vi "Turn And Shoot.vi"(10 "Turning Angle":dbl, 11 "RobotDriveDevRef":T1) -> ()   [LabVIEW 2015]
uses:
  <vilib>/Rock Robotics/WPI/RobotDrive/WPI_RobotDriveArcadeDrive_Standard(NoSaturation).vi
  <vilib>/addons/control/pid/NI_PID_pid.lvlib
  <vilib>/addons/control/pid/pid.llb/PID (DBL).vi
  <vilib>/Rock Robotics/Network Tables/NT Read Number.vi
  <vilib>/Rock Robotics/Network Tables/NT Write Number.vi
  arm/arm.lvclass
  drive/drive.lvclass
  <vilib>/Rock Robotics/WPI/CAN/Jaguar/SubVIs/WPI_CANJaguar_ControlMode.ctl
  <vilib>/Rock Robotics/WPI/CAN/TalonSRX/WPI_CANTalonSRX_APIControlMode.ctl
  <vilib>/Rock Robotics/SystemInterfaces/DIO/FPGA_DIOPWMChannel.ctl
  <vilib>/Rock Robotics/WPI/PWM/WPI_PWMDeadband.ctl
  <vilib>/Rock Robotics/WPI/MotorControl/WPI_MotorControlType.ctl
  <vilib>/Rock Robotics/WPI/MotorControl/WPI_MotorControlDeviceRef.ctl
  <vilib>/Rock Robotics/WPI/RobotDrive/WPI_RobotDriveDevRef.ctl
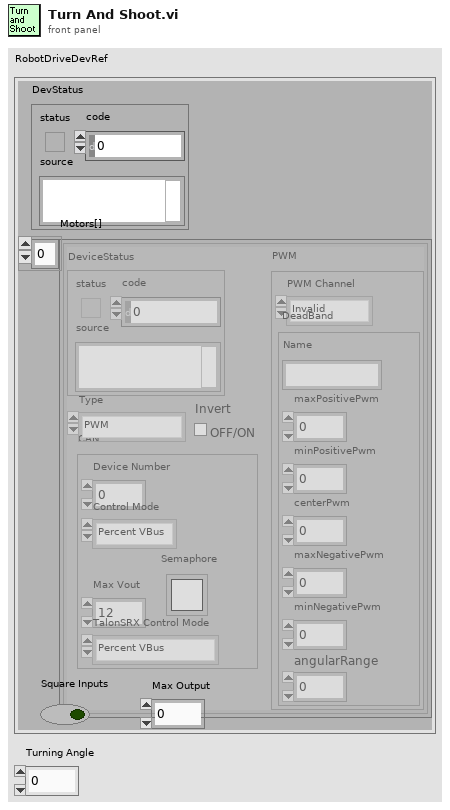
[diagram p1: front panel]
types:
  T1 = typedef "WPI_RobotDriveDevRef.ctl" = cluster{"DevStatus":errorcluster, "Motors[]":T2[], "Square Inputs":bool, "Max Output":dbl}
  T2 = typedef "WPI_MotorControlDeviceRef.ctl" = cluster{"DeviceStatus":errorcluster, "Type":T3, "PWM":cluster{"PWM Channel":T4, "DeadBand":T5}, "CAN":cluster{"Device Number":u8, "Control Mode":T6, "Semaphore":T7, "Max Vout":dbl, "TalonSRX Control Mode":T8}, "Invert":bool}
  T3 = typedef "WPI_MotorControlType.ctl" = enum16{"PWM", "CAN", "CANTalonSRX"}
  T4 = typedef "FPGA_DIOPWMChannel.ctl" = enum8{"PWM 0", "PWM 1", "PWM 2", "PWM 3", "PWM 4", "PWM 5", "PWM 6", "PWM 7", "PWM 8", "PWM 9", "PWM MXP 0", "PWM MXP 1", "PWM MXP 2", "PWM MXP 3", "PWM MXP 4", "PWM MXP 5", "PWM MXP 6", "PWM MXP 7", "PWM MXP 8", "PWM MXP 9", "Invalid"}
  T5 = typedef "WPI_PWMDeadband.ctl" = cluster{"Name":string, "maxPositivePwm":i32, "minPositivePwm":i32, "centerPwm":i32, "maxNegativePwm":i32, "minNegativePwm":i32, "angularRange":u16}
  T6 = typedef "WPI_CANJaguar_ControlMode.ctl" = enum8{"Percent VBus", "Current", "Speed", "Position", "Voltage"}
  T7 = typedef "Semaphore RefNum" = refnum<k1>
  T8 = typedef "WPI_CANTalonSRX_APIControlMode.ctl" = enum8{"Percent VBus", "Speed", "Position", "Slave", "Unchanged / Invalid", "Voltage Compensation", "Current", "Motion Profile"}
  T9 = cluster{"proportional gain (Kc)":dbl, "integral time (Ti, min)":dbl, "derivative time (Td, min)":dbl}
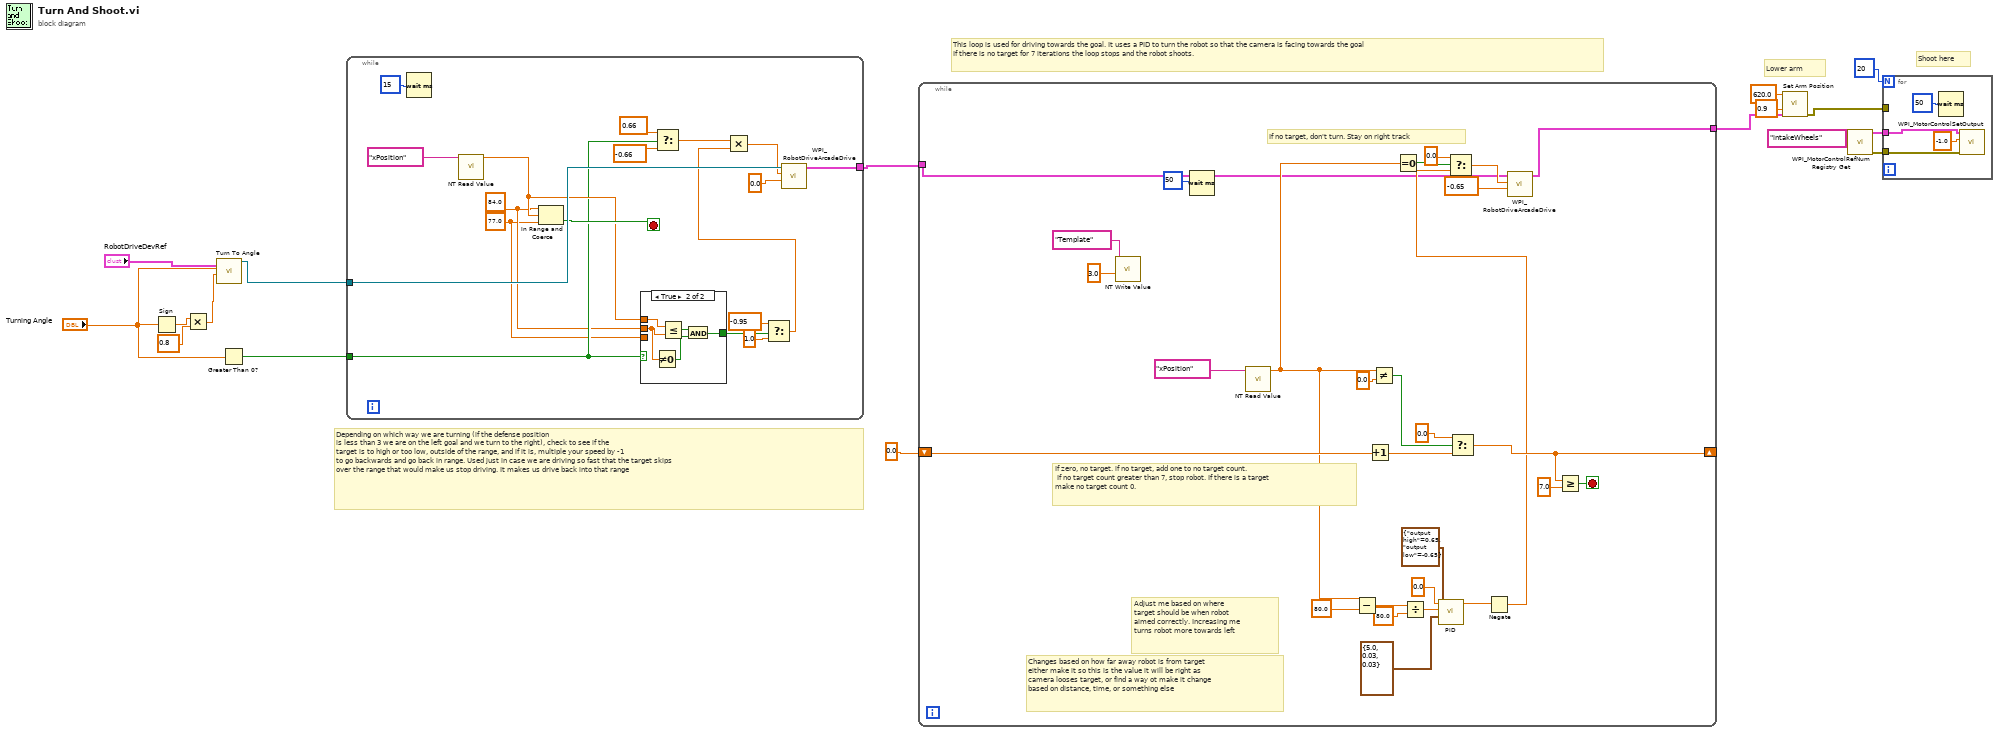
[diagram p0: block diagram]
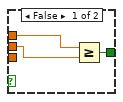
[diagram p2: hidden frame]
diagram:
  # "Depending on which way we are turning (if the defense position \nis less than 3 we are on the left goal and we turn to the right), check to see if the\ntarget is to high or too low, outside of the range, and if it is, multiple your speed by -1\nto go backwards and go back in range. Used just in case we are driving so fast that the target skips\nover the range that would make us stop driving. It makes us drive back into that range"
  # "Lower arm"
  # "This loop is used for driving towards the goal. It uses a PID to turn the robot so that the camera is facing towards the goal\nIf there is no target for 7 iterations the loop stops and the robot shoots."
  # "Shoot here"
  n1 = Sign(1:"Turning Angle") -> (0:w14:dbl)
  n2 = Multiply(x=w14, y=0.8) -> (x*y=w16:dbl)
  n3 = call "Turn To Angle.vi"(7:"RobotDriveDevRef", "Speed/Direction"=w16, "Angle"="Turning Angle") -> ("drive.lvclass"=w13:refnum<class "drive.lvclass">)  [unwired: 7 in, 1 out]
  n4 = Greater Than 0?(x="Turning Angle") -> (x > 0?=w5:bool)
  n5 = while {
    tunnel: [w33] -> w3
    tunnel: w13 -> [w32]
    tunnel: w5 -> [w20]
    stop <- w30 stop-if-true
    w18 = 77.0 ("lower limit")
    w19 = 84.0 ("upper limit")
    n6 = Wait (ms)(milliseconds to wait=u32 15) -> ()  [unwired: 1 out]
    n7 = call-poly <vilib>:"NT Read Value.vi"("Name"="xPosition") -> ("Numeric"=w21:dbl)  [unwired: 9 in, 1 out]
    n8 = In Range and Coerce(upper limit=w19, x=w21, lower limit=w18) -> (In Range?=w30:bool)  [unwired: 1 out]
    n9 = case shown="True" w20 {
      tunnel: w19 -> [w37 w40]
      tunnel: w18 -> [_ _]
      tunnel: [w38 w41] -> w26
      tunnel: w21 -> [w36 w39]
      frame False {
        n10 = Greater Or Equal?(x=w36, y=w37) -> (x >= y?=w38:bool)
      }
      frame True {
        n11 = Not Equal To 0?(x=w40) -> (x != 0?=w42:bool)
        n12 = Less Or Equal?(x=w39, y=w40) -> (x <= y?=w43:bool)
        n13 = And(x=w43, y=w42) -> (x .and. y?=w41:bool)
      }
    }
    n14 = Select(t=0.66, s=w20, f=-0.66) -> (s? t:f=w27:dbl)
    n15 = Select(t=-0.95, s=w26, f=1.0) -> (s? t:f=w23:dbl)
    n16 = Multiply(x=w27, y=w23) -> (x*y=w22:dbl)
    n17 = call-poly <vilib>:"WPI_RobotDriveArcadeDrive.vi"("Y axis value"=0.0, "X axis value"=w22, "RobotDriveDevRef"=w32) -> ("RobotDriveDevRef"=w33:T1)  [unwired: 6 in, 2 out]
  }
  n18 = while {
    shift-right: [w59] -> _
    shift-left: 0.0 ("t") -> [w62]
    tunnel: [w64] -> w1
    tunnel: w3 -> [w44]
    stop <- w48 stop-if-true
    # "Changes based on how far away robot is from target\neither make it so this is the value it will be right as\ncamera looses target, or find a way ot make it change\nbased on distance, time, or something else"
    # "Adjust me based on where\ntarget should be when robot\naimed correctly. Increasing me\nturns robot more towards left"
    # "If no target, don't turn. Stay on right track"
    # "If zero, no target. if no target, add one to no target count.\n If no target count greater than 7, stop robot. If there is a target\nmake no target count 0."
    n19 = call-poly <vilib>:"NT Write Value.vi"("Numeric"=3.0, "Name"="Template") -> ()  [unwired: 9 in, 1 out]
    n20 = Wait (ms)(milliseconds to wait=u32 50) -> ()  [unwired: 1 out]
    n21 = call-poly <vilib>:"NT Read Value.vi"("Name"="xPosition") -> ("Numeric"=w47:dbl)  [unwired: 9 in, 1 out]
    n22 = Subtract(x=w47, y=80.0) -> (x-y=w53:dbl)
    n23 = Increment(x=w62) -> (x+1=w61:dbl)
    n24 = Not Equal?(x=w47, y=0.0) -> (x != y?=w63:bool)
    n25 = Equal To 0?(x=w47) -> (x = 0?=w57:bool)
    n26 = Divide(x=w53, y=80.0) -> (x/y=w49:dbl)
    n27 = call-poly <vilib>:"PID.vi"("output range"=cluster{"output high":dbl, "output low":dbl} {"output high"=0.65, "output low"=-0.65}, "PID gains"=T9 {"proportional gain (Kc)"=5.0, "integral time (Ti, min)"=0.03, "derivative time (Td, min)"=0.03} ("Turn robot to camera 2"), "process variable"=w49, "setpoint"=0.0) -> ("output"=w67:dbl)  [unwired: 6 in, 1 out]
    n28 = Select(t=0.0, s=w63, f=w61) -> (s? t:f=w59:dbl)
    n29 = Negate(x=w67) -> (-x=w46:dbl)
    n30 = Select(t=0.0, s=w57, f=w46) -> (s? t:f=w55:dbl)
    n31 = call-poly <vilib>:"WPI_RobotDriveArcadeDrive.vi"("Y axis value"=-0.65 ("f"), "X axis value"=w55, "RobotDriveDevRef"=w44) -> ("RobotDriveDevRef"=w64:T1)  [unwired: 6 in, 2 out]
    n32 = Greater Or Equal?(x=w59, y=7.0) -> (x >= y?=w48:bool)
  }
  n33 = call "Set Arm Position.vi"("error in (no error)"=w1, "Setpoint"=0.9 ("Speed"), "arm.lvclass"=620.0 ("Setpoint")) -> ("error out (no error)"=w6:errorcluster)  [unwired: 7 in, 1 out]
  n34 = call <vilib>:"WPI_MotorControlRefNum Registry Get.vi"("refnum name"="intakeWheels") -> ("error out"=w9:errorcluster, "MotorControlDevRef"=w10:T2)  [unwired: 9 in]
  n35 = for {
    N: 20 -> [_]
    tunnel: w9 -> [w75]
    tunnel: w10 -> [w74]
    tunnel: w6 -> [_]
    n36 = Wait (ms)(milliseconds to wait=u32 50) -> ()  [unwired: 1 out]
    n37 = call <vilib>:"WPI_MotorControlSetOutput.vi"("error in (no error)"=w75, "Output"=-1.0, "MotorControlDevRef"=w74) -> ()  [unwired: 6 in, 3 out]
  }
